vi "Technician Global.vi"(7 "Write? (F)":bool, 11 "Technician Name":string) -> (3 "Technician Name":string)   [LabVIEW 2019]
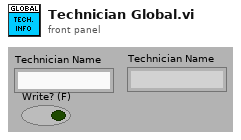
[diagram p1: front panel]
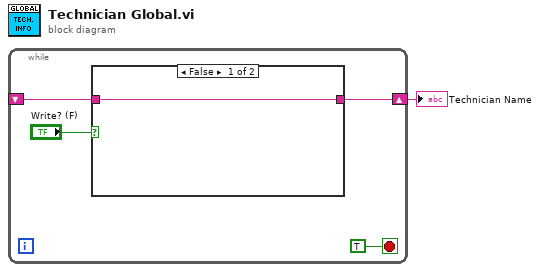
[diagram p0: block diagram]
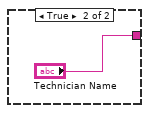
[diagram p2: hidden frame]
diagram:
  n1 = while {
    shift-right: [w3] -> w1
    shift-left: _ -> [w2]
    stop <- TRUE stop-if-true
    n2 = case shown="False" "Write? (F)" {
      tunnel: [w6 "Technician Name"] -> w3
      tunnel: w2 -> [w6 _]
      frame False {
      }
      frame True {
      }
    }
  }
  "Technician Name" <- w1
